vi "IO_DataQ_Read_All.vi"(8 "error in (no error)":errorcluster, 10 "Bytes at Port":u32, 11 "VISA Refnum in":refnum<visa-resource-name>) -> (0 "error out":errorcluster, 1 "Dout":i16 format="%x", 2 "Aout":dbl[][](array[numeric]), 3 "VISA Refnum out":refnum<visa-resource-name>)   [LabVIEW 2024]
panel:
  out "Chart":dbl[][](graph)
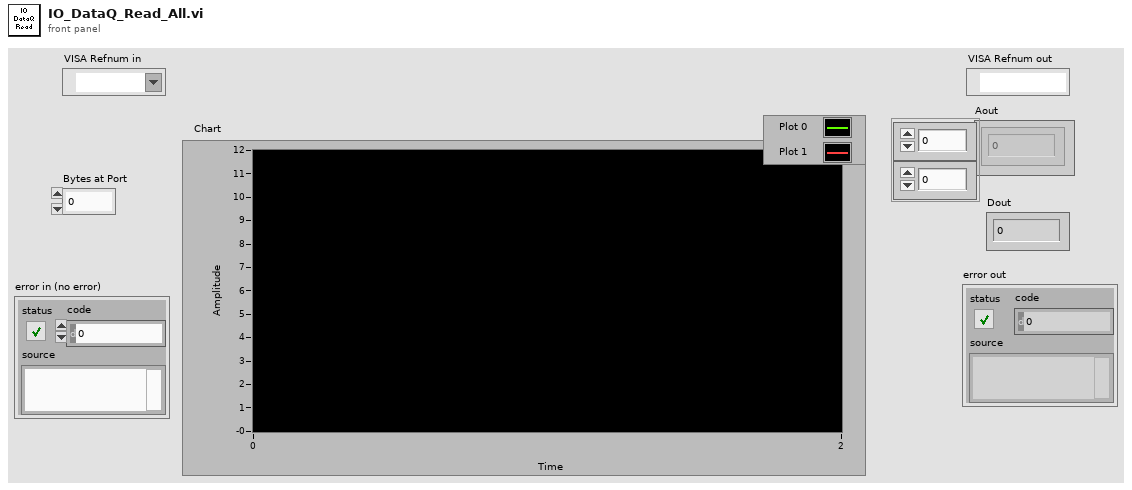
[diagram p1: front panel]
types:
  T1 = enum16{"big-endian, network order", "native, host order", "little-endian"}
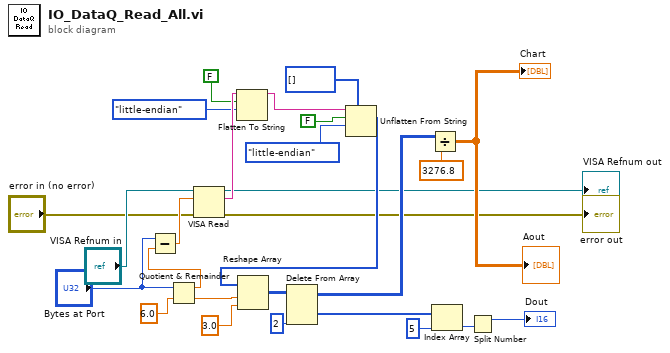
[diagram p0: block diagram]
diagram:
  n1 = Quotient & Remainder(x="Bytes at Port", y=6.0) -> (x-y*floor(x/y)=w27:dbl, floor(x/y)=w16:dbl)
  n2 = Subtract(x="Bytes at Port", y=w27) -> (x-y=w5:dbl)
  n3 = VISA Read(VISA resource name="VISA Refnum in", byte count=w5, error in (no error)="error in (no error)") -> (VISA resource name out=→"VISA Refnum out":refnum<visa-resource-name>, read buffer=w13:string, error out=→"error out":errorcluster)  [unwired: 1 out]
  n4 = Flatten To String(anything=w13, prepend array or string size? (T)=FALSE, byte order (0:big-endian, network order)=T1."little-endian") -> (data string=w12:string)  [unwired: 1 in, 2 out]
  n5 = Unflatten From String(type=i16[] [], binary string=w12, data includes array or string size? (T)=FALSE, byte order (0:big-endian, network order)=T1."little-endian") -> (value=w18:i16[])  [unwired: 1 in, 2 out]
  n6 = Reshape Array(w18, w16, 3.0) -> (w20:i16[][])
  n7 = Delete From Array(array=w20, index (col)=2 ("disabled index (col)")) -> (deleted portion=w23:i16[], array with subset deleted=w22:i16[][])  [unwired: 2 in]
  n8 = Divide(x=w22, y=3276.8) -> (x/y=→"Chart" →"Aout":dbl[][])
  n9 = Index Array(array=w23, index=5 ("disabled index (row)")) -> (element=w24:i16)
  n10 = Split Number(x=w24) -> (hi(x)=→"Dout":u8)  [unwired: 1 out]
